vi "Apply Strings and Values.vi"(8 "error in (no error)":errorcluster, 11 "Dynamic Combobox in":refnum<class "Dynamic Combobox.lvclass">) -> (0 "error out":errorcluster, 3 "Dynamic Combobox out":refnum<class "Dynamic Combobox.lvclass">)   [LabVIEW 2020, in "Dynamic Combobox.lvlib" / "Dynamic Combobox.lvclass"]
uses:
  Dynamic Combobox.lvclass
  Dynamic Combobox.lvclass/Dynamic Combobox.ctl
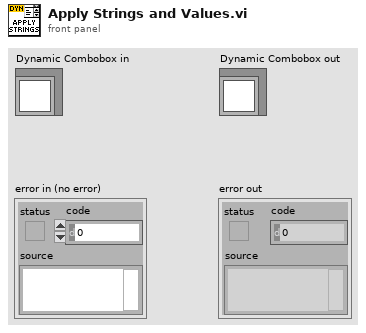
[diagram p1: front panel]
types:
  T1 = typedef "Dynamic Combobox.lvlib/Dynamic Combobox.lvclass/Ref Data.ctl" = cluster{"Values":refnum<class "Dynamic Values.lvclass">, "Debug":bool, "Strings And Values []":T2, "Options":T3}
  T2 = typedef "LVComboBoxStrsAndValuesArrayTypeDef.ctl" = cluster{"String":string, "Value":string}[]
  T3 = typedef "Dynamic Combobox.lvlib/Dynamic Combobox.lvclass/Options.ctl" = cluster{"Browse Entry":bool, "Refresh Entry":bool, "Allow Undefined Values":bool}
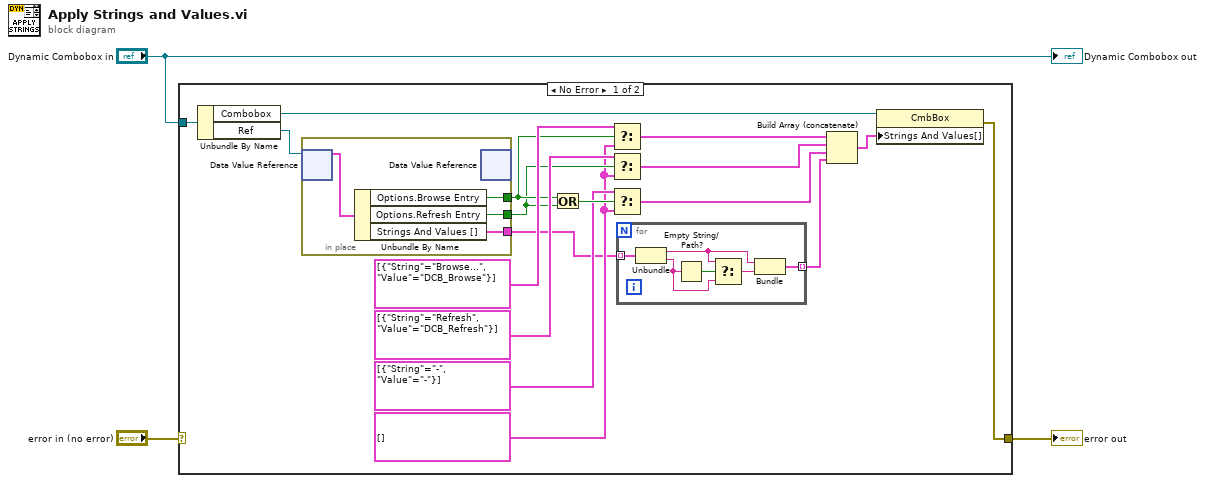
[diagram p0: block diagram]
diagram:
  n1 = case shown="No Error" "error in (no error)" {
    selector: "error in (no error)" -> [_ w31]
    tunnel: "Dynamic Combobox in" -> [w7 _]
    tunnel: [w6 w31] -> w1
    frame No Error {
      w13 = cluster{"String":string, "Value":string}[] []
      n2 = Unbundle By Name(w7) -> ("Combobox"=w9:refnum<vi>, "Ref"=w20:refnum<data-value>)
      n3 = in-place {
        in-place-border: [w29] -> w5
        in-place-border: [w28] -> w17
        in-place-border: [w27] -> w16
        n4 = in-place-dvr #1(w20) -> (w30:T1)  [unwired: 1 out]
        n5 = Unbundle By Name(w30) -> ("Options.Browse Entry"=w28:bool, "Options.Refresh Entry"=w27:bool, "Strings And Values []"=w29:T2)
        n6 = in-place-dvr #1() -> ()  [unwired: 1 in, 2 out]
      }
      n7 = Or(x=w17, y=w16) -> (x .or. y?=w15:bool)
      n8 = Select(t=cluster{"String":string, "Value":string}[] [{"String"="Browse...", "Value"="DCB_Browse"}], s=w17, f=w13) -> (s? t:f=w10:cluster{"String":string, "Value":string}[])
      n9 = Select(t=cluster{"String":string, "Value":string}[] [{"String"="Refresh", "Value"="DCB_Refresh"}], s=w16, f=w13) -> (s? t:f=w11:cluster{"String":string, "Value":string}[])
      n10 = Select(t=cluster{"String":string, "Value":string}[] [{"String"="-", "Value"="-"}], s=w15, f=w13) -> (s? t:f=w12:cluster{"String":string, "Value":string}[])
      n11 = for {
        tunnel: w5 -> [w26] mode=indexing
        tunnel: [w21] -> w4 mode=indexing
        n12 = Unbundle(w26) -> ("String"=w22:string, "Value"=w24:string)
        n13 = Empty String/Path?(string/path=w24) -> (empty?=w25:bool)
        n14 = Select(t=w22, s=w25, f=w24) -> (s? t:f=w23:string)
        n15 = Bundle("String"=w22, "Value"=w23) -> (w21:cluster{"String":string, "Value":string})  [unwired: 1 in]
      }
      n16 = Build Array (concatenate)(w10, w11, w12, w4) -> (w8:cluster{"String":string, "Value":string}[])
      n17 = property class="CmbBox"(reference=w9, "Strings And Values[]"=w8) -> (error out=w6:errorcluster)  [unwired: 1 in, 1 out]
    }
    frame Error {
    }
  }
  "error out" <- w1
  "Dynamic Combobox out" <- "Dynamic Combobox in"
